vi "Log String.vi"(5 "String":string, 7 "Level":T1, 8 "error in (no error)":errorcluster) -> (0 "error out":errorcluster)   [LabVIEW 2016, in "Stream Log.lvlib" / "Global Application Log.lvclass"]
doc: "--\nCopyright © 2017 Composed SystemsI All rights reserved.\n\nAuthor: Jon McBee <jon.mcbee@composed.io>\n\nThis library is provided \"AS IS\" ,WITHOUT WARRANTIES OR\nCONDITIONS OF ANY KIND, either express or implied.\n\nComposed Systems -- composed.io\n\nStream 0.0.1.1\nJon McBee - Composed Systems\nCopyright (c) 2017, Composed Systems"
uses:
  <userlib>/Composed Systems/Stream/Log/Global Application Log/Global Application Log.lvclass
  <userlib>/Composed Systems/Stream/Log/Application Log/Log Level.ctl
  <userlib>/Composed Systems/Stream/Log/Global Application Log/Global Application Log.lvclass/Global Application Log.ctl
  <userlib>/Composed Systems/Stream/Log/Application Log/Application Log.lvclass
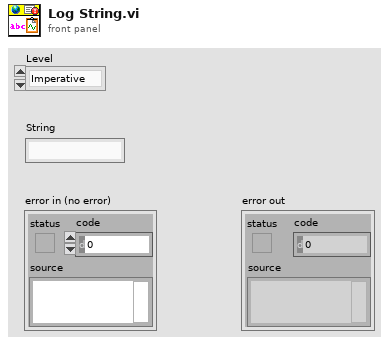
[diagram p1: front panel]
types:
  T1 = typedef "Stream Log.lvlib/Application Log.lvclass/Log Level.ctl" = enum16{"Imperative", "Major", "Minor", "Debug", "Off"}
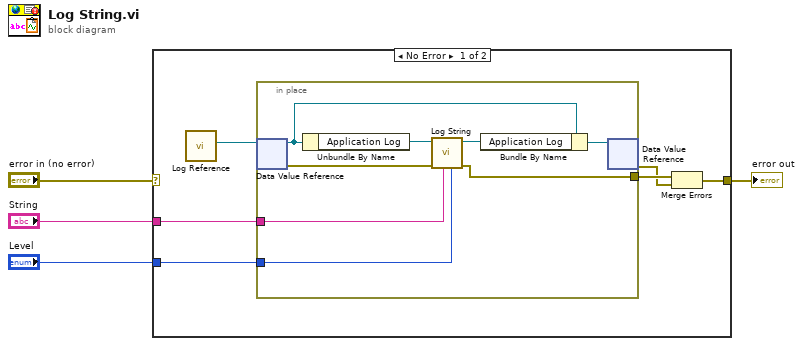
[diagram p0: block diagram]
diagram:
  n1 = case shown="No Error" "error in (no error)" {
    selector: "error in (no error)" -> [_ w19]
    tunnel: [w5 w19] -> w3
    tunnel: "String" -> [w9 _]
    tunnel: "Level" -> [w8 _]
    frame No Error {
      n2 = call <userlib>:"Log Reference.vi"() -> ("Global Log Reference out"=w10:refnum<data-value>)  [unwired: 11 in]
      n3 = in-place {
        in-place-border: w9 -> [w18]
        in-place-border: w8 -> [w17]
        in-place-border: [w11] -> w7
        n4 = in-place-dvr #1(w10) -> (w15:refnum<class "Global Application Log.lvclass">, w12:errorcluster)
        n5 = Unbundle By Name(w15) -> ("Application Log"=w16:refnum<class "Application Log.lvclass">)
        n6 = call-dynamic "Log String.vi"("Level"=w17, "String"=w18, "error in (no error)"=w12, "Application Log in"=w16) -> ("error out"=w11:errorcluster, "Application Log out"=w14:refnum<class "Application Log.lvclass">)  [unwired: 6 in]
        n7 = Bundle By Name(cluster=w15, "Application Log"=w14) -> (w13:refnum<class "Global Application Log.lvclass">)
        n8 = in-place-dvr #1(w13) -> (w6:errorcluster)  [unwired: 1 out]
      }
      n9 = Merge Errors(w7, w6) -> (w5:errorcluster)
    }
    frame Error {
    }
  }
  "error out" <- w3
